vi "BezierGenerator.vi"(0 "DeltaX":dbl=60.0, 1 "DeltaY":dbl=60.0, 2 "TargetName":string, 3 "RobotOrientation":dbl=70.0, 4 "Image In":T1) -> (5 "SmoothedPath":cluster{"x":dbl, "y":dbl}[](array[cluster]))   [LabVIEW 2018]
uses:
  <vilib>/vision/Image Controls.llb/IMAQ Image.ctl
panel:
  out "CurvePoints":cluster{"x":dbl, "y":dbl}[](array[cluster])
  out "Path Drawer":T1(plugin-control)
  out "waypoints":cluster{dbl[], dbl[]}(graph)
  in  "TrajPointoffset":dbl=12.0
  in  "TargetOffset":dbl=12.0
  out "Curve":cluster{"X":dbl, "Y":dbl}[](graph)
  in  "Path":cluster{"x":dbl, "y":dbl}[](array[cluster])=[{"x"=0.0, "y"=0.0}, {"x"=0.0, "y"=0.0}, {"x"=0.0, "y"=0.0}, {"x"=0.0, "y"=0.0}]
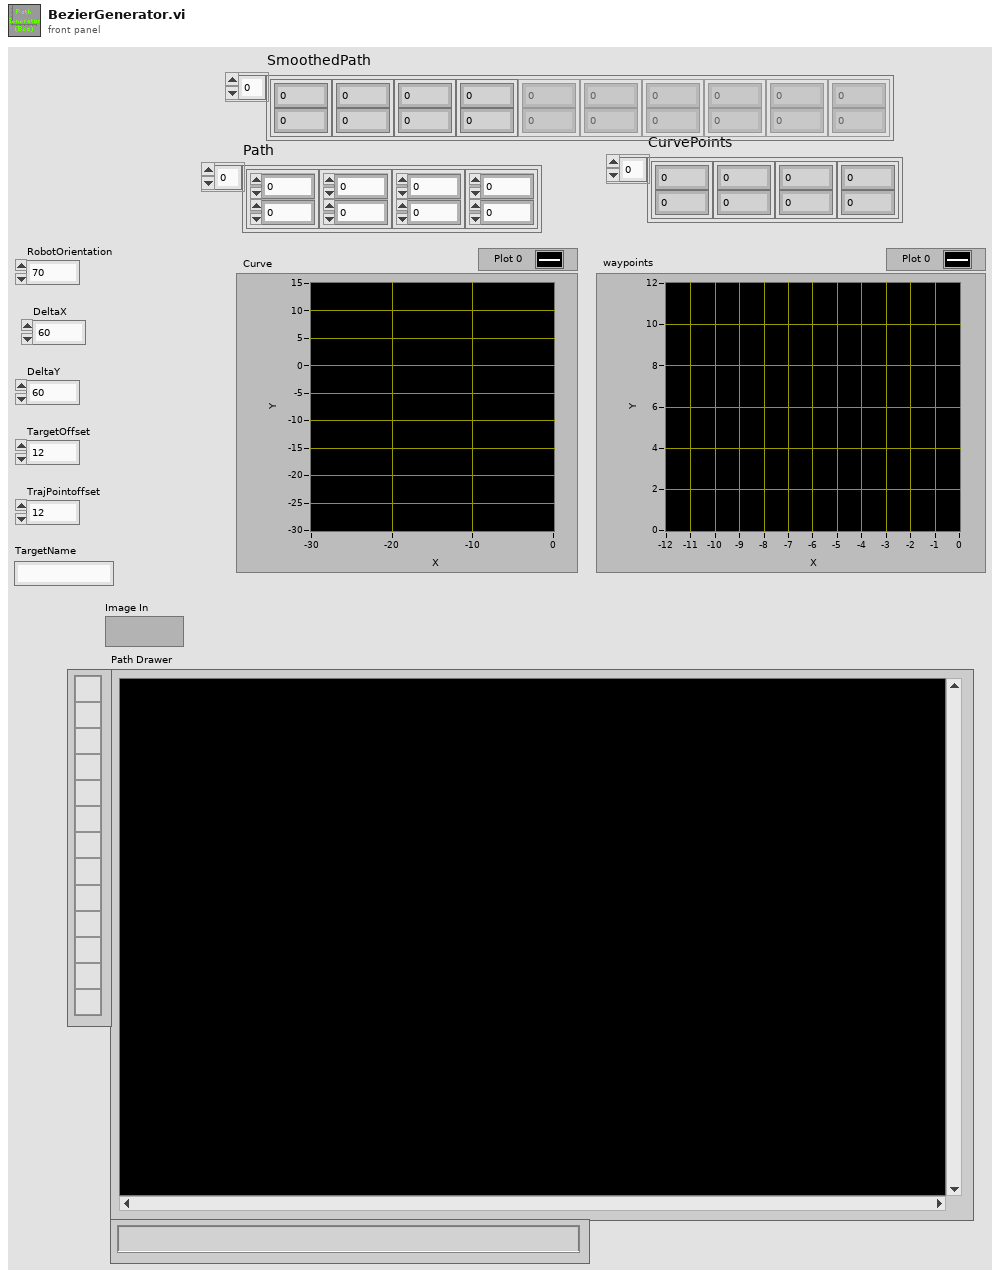
[diagram p1: front panel]
types:
  T1 = typedef "IMAQ Image.ctl" = refnum<image>
  T2 = typedef "TargetDataType.ctl" = cluster{"Name":string, "x":dbl, "y":dbl, "orientation":dbl, "height":dbl}
  T3 = cluster{"Target":T2, "DeltaX":dbl, "DeltaY":dbl, "RobotOrientation":dbl, "TrajPointoffset":dbl, "TargetOffset":dbl}
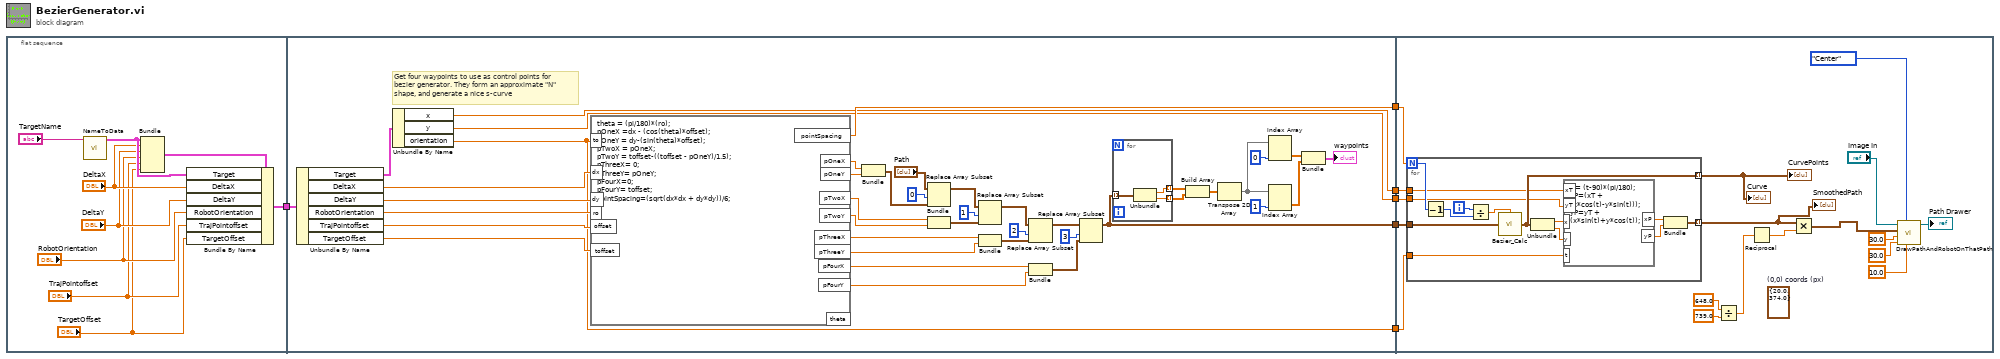
[diagram p0: block diagram]
diagram:
  n1 = flat-sequence {
    tunnel: [w13] -> w4
    tunnel: [w38] -> w6
    tunnel: [w25] -> w5
    tunnel: w4 -> [w32]
    tunnel: [w18] -> w3
    tunnel: [w17] -> w2
    tunnel: [w16] -> w1
    tunnel: w6 -> [w77]
    tunnel: w5 -> [w69]
    tunnel: w3 -> [w67]
    tunnel: w2 -> [w66]
    tunnel: w1 -> [w65]
    frame #0 {
      n2 = call "NameToData.vi"("Name"="TargetName") -> ("Target"=w12:T2)  [unwired: 10 in]
      n3 = Bundle("Target"=w12, "DeltaX"="DeltaX", "DeltaY"="DeltaY", "RobotOrientation"="RobotOrientation", "TrajPointoffset"="TrajPointoffset", "TargetOffset"="TargetOffset") -> (w14:T3)  [unwired: 1 in]
      n4 = Bundle By Name(cluster=w14, "Target"=w12, "DeltaX"="DeltaX", "DeltaY"="DeltaY", "RobotOrientation"="RobotOrientation", "TrajPointoffset"="TrajPointoffset", "TargetOffset"="TargetOffset") -> (w13:T3)
    }
    frame #1 {
      # "Get four waypoints to use as control points for bezier generator. They form an approximate \"N\" shape, and generate a nice s-curve"
      n5 = Unbundle By Name(w32) -> ("Target"=w29:T2, "DeltaX"=w31:dbl, "DeltaY"=w30:dbl, "RobotOrientation"=w26:dbl, "TrajPointoffset"=w27:dbl, "TargetOffset"=w28:dbl)
      n6 = Unbundle By Name(w29) -> ("x"=w17:dbl, "y"=w16:dbl, "orientation"=w18:dbl)
      n7 = formula code="theta = (pi/180)*(ro);\npOneX =dx - (cos(theta)*offset);\npOneY = dy-(sin(theta)*offset);\npTwoX = pOneX;\npTwoY = toffset-((toffset - pOneY)/1.5);\npThreeX= 0;\npThreeY= pOneY;\npFourX=0;\npFourY= toffset;\npointSpacing=(sqrt(dx*dx + dy*dy))/6;"("ro"=w26, "dx"=w31, "dy"=w30, "to"=w18, "offset"=w27, "toffset"=w28) -> ("pOneX"=w36:dbl, "pOneY"=w35:dbl, "pTwoX"=w34:dbl, "pTwoY"=w33:dbl, "pointSpacing"=w25:dbl, "pThreeX"=w24:dbl, "pThreeY"=w23:dbl, "pFourX"=w22:dbl, "pFourY"=w21:dbl)  [unwired: 1 out]
      n8 = Bundle("pOneX"=w36, "pOneY"=w35) -> (w47:cluster{"pOneX":dbl, "pOneY":dbl})  [unwired: 1 in]
      n9 = Replace Array Subset(array="Path", new element=w47, index=0) -> (w53:cluster{"x":dbl, "y":dbl}[])
      n10 = Bundle("pTwoX"=w34, "pTwoY"=w33) -> (w48:cluster{"pTwoX":dbl, "pTwoY":dbl})  [unwired: 1 in]
      n11 = Replace Array Subset(array=w53, new element=w48, index=1) -> (w51:cluster{"x":dbl, "y":dbl}[])
      n12 = Bundle("pThreeX"=w24, "pThreeY"=w23) -> (w19:cluster{"pThreeX":dbl, "pThreeY":dbl})  [unwired: 1 in]
      n13 = Replace Array Subset(array=w51, new element=w19, index=2) -> (w49:cluster{"x":dbl, "y":dbl}[])
      n14 = Bundle("pFourX"=w22, "pFourY"=w21) -> (w20:cluster{"pFourX":dbl, "pFourY":dbl})  [unwired: 1 in]
      n15 = Replace Array Subset(array=w49, new element=w20, index=3) -> (w38:cluster{"x":dbl, "y":dbl}[])
      n16 = for {
        tunnel: w38 -> [w59] mode=indexing
        tunnel: [w58] -> w46 mode=indexing
        tunnel: [w57] -> w45 mode=indexing
        n17 = Unbundle(w59) -> ("x"=w58:dbl, "y"=w57:dbl)
      }
      n18 = Build Array(w46, w45) -> (w44:dbl[][])
      n19 = Transpose 2D Array(2D array=w44) -> (transposed array=w41:dbl[][])
      n20 = Index Array(array=w41, index (col)=0 ("disabled index (col)")) -> (element=w39:dbl[])  [unwired: 1 in]
      n21 = Index Array(array=w41, index (col)=1 ("disabled index (col)")) -> (element=w40:dbl[])  [unwired: 1 in]
      n22 = Bundle(w39, w40) -> (→"waypoints":cluster{dbl[], dbl[]})  [unwired: 1 in]
    }
    frame #2 {
      (unwired) cluster{dbl, dbl} {20.0, 374.0}  # (0,0) coords (px)
      n23 = for {
        N: w69 -> [w91]
        tunnel: [w84] -> w61 mode=indexing
        tunnel: w77 -> [w87]
        tunnel: [w81] -> w64 mode=indexing
        tunnel: w67 -> [w80]
        tunnel: w66 -> [w79]
        tunnel: w65 -> [w78]
        i -> [w90]
        n24 = Decrement(x=w91) -> (x-1=w89:i32)
        n25 = Divide(x=w90, y=w89) -> (x/y=w88:dbl)
        n26 = call "Bezier_Calc.vi"("points"=w87, "t"=w88) -> ("point out"=w81:cluster{"x":dbl, "y":dbl})
        n27 = Unbundle(w81) -> ("x"=w83:dbl, "y"=w82:dbl)
        n28 = formula code="t = (t-90)*(pi/180);\nxP=(xT + (x*cos(t)-y*sin(t)));\nyP=yT + (x*sin(t)+y*cos(t));"("x"=w83, "y"=w82, "t"=w80, "xT"=w79, "yT"=w78) -> ("yP"=w85:dbl, "xP"=w86:dbl)
        n29 = Bundle("xP"=w86, "yP"=w85) -> (w84:cluster{"xP":dbl, "yP":dbl})  [unwired: 1 in]
      }
      "Curve" <- w64
      "CurvePoints" <- w64
      "SmoothedPath" <- w61
      n30 = Divide(x=648.0, y=739.0) -> (x/y=w68:dbl)
      n31 = Reciprocal(x=w68) -> (1/x=w63:dbl)
      n32 = Multiply(x=w61, y=w63) -> (x*y=w62:cluster{"xP":dbl, "yP":dbl}[])
      n33 = call "DrawPathAndRobotOnThatPath.vi"("CenterOfRotYOffset (px)"=10.0, "PathMode"=enum16{"Left", "Right", "Center"}."Center", "RobotLength (px)"=30.0, "RobotWidth (px)"=30.0, "Path (px)"=w62, "Image In"="Image In") -> ("Image Out"=→"Path Drawer":T1)  [unwired: 4 in, 1 out]
    }
  }
